vi "cook.vi"(8 "error in (no error)":errorcluster, 11 "Bake in":refnum<class "Bake.lvclass">) -> (0 "error out":errorcluster, 3 "Bake out":refnum<class "Bake.lvclass">)   [LabVIEW 2010, in "CookBehaviors.lvlib" / "Bake.lvclass"]
uses:
  Bake.lvclass
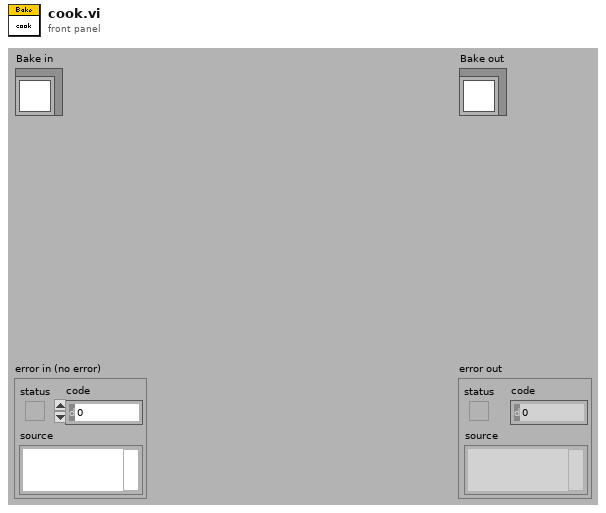
[diagram p1: front panel]
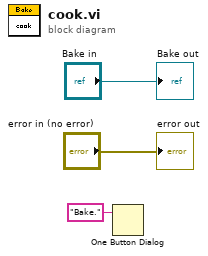
[diagram p0: block diagram]
diagram:
  n1 = One Button Dialog(message="Bake.") -> ()  [unwired: 1 in, 1 out]
  "error out" <- "error in (no error)"
  "Bake out" <- "Bake in"
